vi "State Set Digital Output.vi"(8 "Sys Error In":errorcluster, 9 "task/channels in":refnum<k21> caption="任务/通道输入", 10 "Step Description":string, 11 "Step Data String":string) -> (0 "Sys Error Out":errorcluster, 1 "Error No.":u16, 2 "Error String":string, 3 "Pass?":bool)   [LabVIEW 2018]
uses:
  05.UserVI's/type defs/EOL Global Digital Output Cluster Control.ctl
  05.UserVI's/type defs/EOL Global Digital Output Control.ctl
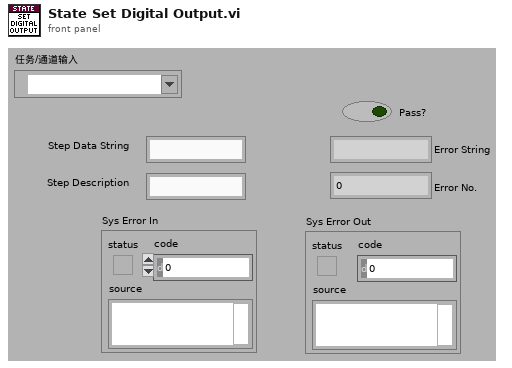
[diagram p1: front panel]
types:
  T1 = enum16{"Init", "Write", "Write All", "Clear All", "Stop"}
  T2 = typedef "EOL Global Digital Output Cluster Control.ctl" = cluster{"Status":bool, "Global DO Ch":T3}
  T3 = typedef "EOL Global Digital Output Control.ctl" = enum16{"Battery", "IGN High", "IGN Low", "LIN", "CAN", "Switch 1", "Switch 2", "Switch 3", "Switch 4", "Switch 5", "Switch 6", "Glass Analog Switch 1", "Glass Analog Switch 2", "Glass Analog Switch 3", "Glass Analog Switch 4", "Sunshade Analog Switch 1", "Sunshade Analog Switch 2", "Sunshade Analog Switch 3", "Sunshade Analog Switch 4", "Glass Motor Relay 1", "Glass Motor Relay 2", "Sunshade Motor Relay 1", "Sunshade Motor Relay 2"}
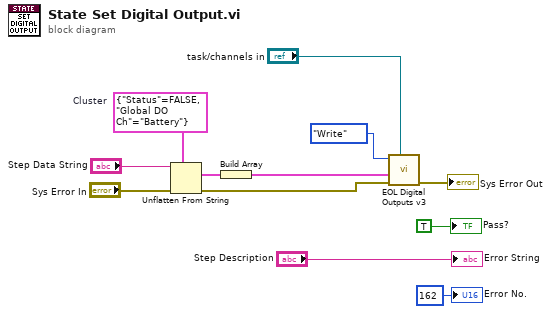
[diagram p0: block diagram]
diagram:
  w11 = T2 {"Status"=FALSE, "Global DO Ch"=enum."Battery"}  # Cluster
  n1 = Unflatten From String(type=w11, binary string="Step Data String", error in (no error)="Sys Error In") -> (value=w3:T2, error out=w9:errorcluster)  [unwired: 2 in, 1 out]
  n2 = Build Array(w3) -> (w2:T2[])
  n3 = call "EOL Digital Outputs v3.vi"("task/channels in"="task/channels in", "Error In"=w9, "DO Status"=w2, "Mode"=T1."Write") -> ("Error Out"=→"Sys Error Out":errorcluster)  [unwired: 6 in, 1 out]
  "Error String" <- "Step Description"
  "Error No." <- u16 162 ("Error No.")
  "Pass?" <- TRUE ("Pass?")
